vi "led state.vi"() -> ()   [LabVIEW 2019]
panel:
  out "Boolean 3":bool
  out "Boolean 2":bool
  out "Boolean":bool
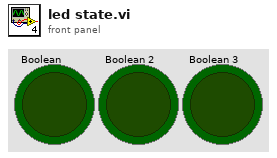
[diagram p1: front panel]
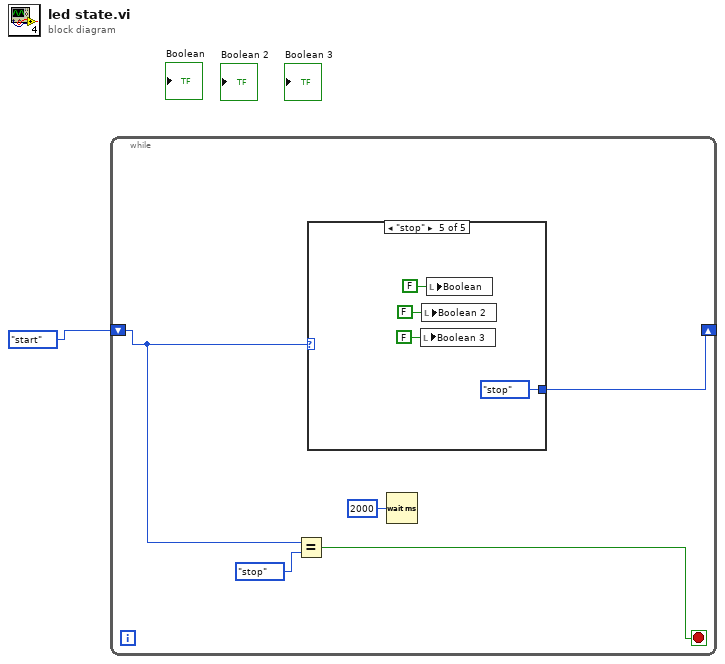
[diagram p0: block diagram]
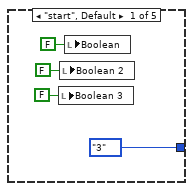
[diagram p2: hidden frame]
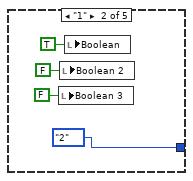
[diagram p3: hidden frame]
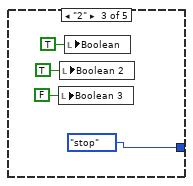
[diagram p4: hidden frame]
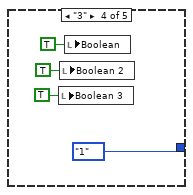
[diagram p5: hidden frame]
diagram:
  n1 = while {
    shift-right: [w6] -> _
    shift-left: enum16{"start", "1", "2", "3", "stop"}."start" ("Enum") -> [w4]
    stop <- w2 stop-if-true
    n2 = Equal?(x=w4, y=enum16{"start", "1", "2", "3", "stop"}."stop" ("Enum")) -> (x = y?=w2:bool)
    n3 = case shown="\"stop\"" w4 {
      tunnel: [enum16{"start", "1", "2", "3", "stop"}."3" ("Enum") enum16{"start", "1", "2", "3", "stop"}."2" ("Enum") enum16{"start", "1", "2", "3", "stop"}."stop" ("Enum") enum16{"start", "1", "2", "3", "stop"}."1" ("Enum") enum16{"start", "1", "2", "3", "stop"}."stop" ("Enum")] -> w6
      frame "start", Default {
        n4 = local write "Boolean 3"(FALSE ("Boolean 3")) -> ()
        n5 = local write "Boolean 2"(FALSE ("Boolean 2")) -> ()
        n6 = local write "Boolean"(FALSE ("Boolean")) -> ()
      }
      frame "1" {
        n7 = local write "Boolean 3"(FALSE ("Boolean 3")) -> ()
        n8 = local write "Boolean 2"(FALSE ("Boolean 2")) -> ()
        n9 = local write "Boolean"(TRUE ("Boolean")) -> ()
      }
      frame "2" {
        n10 = local write "Boolean 3"(FALSE ("Boolean 3")) -> ()
        n11 = local write "Boolean 2"(TRUE ("Boolean 2")) -> ()
        n12 = local write "Boolean"(TRUE ("Boolean")) -> ()
      }
      frame "3" {
        n13 = local write "Boolean 3"(TRUE ("Boolean 3")) -> ()
        n14 = local write "Boolean 2"(TRUE ("Boolean 2")) -> ()
        n15 = local write "Boolean"(TRUE ("Boolean")) -> ()
      }
      frame "stop" {
        n16 = local write "Boolean 3"(FALSE ("Boolean 3")) -> ()
        n17 = local write "Boolean 2"(FALSE ("Boolean 2")) -> ()
        n18 = local write "Boolean"(FALSE ("Boolean")) -> ()
      }
    }
    n19 = Wait (ms)(milliseconds to wait=u32 2000) -> ()  [unwired: 1 out]
  }
